vi "Lab1.vi"() -> ()   [LabVIEW 2010]
uses:
  <vilib>/measure/maspectr.llb/FFT Spectrum (Mag-Phase) for 1 Chan.vi
  <vilib>/measure/NI_MABase.lvlib
  <vilib>/measure/NI_MAPro.lvlib
  <vilib>/ptbypt/NI_PtbyPt.lvlib
panel:
  out "Power Ratio":dbl
  out "Baseband Signal (Time)":waveform(dbl)(graph)
  out "Baseband Signal (frequency)":cluster{"f0":dbl, "df":dbl, "magnitude":dbl[]}(graph)
  out "Modulated Signal (frequency)":cluster{"f0":dbl, "df":dbl, "magnitude":dbl[]}(graph)
  in  "stop":bool
  in  "Modulation Index":dbl(slide)=1.0 scale=0.0..1.0
  in  "Modulation Freq":dbl(slide)=10.0 scale=0.0..1000.0
  in  "Carrier Freq":dbl(slide)=10.0 scale=0.0..500000.0
  out "Modulated Signal (Time)":waveform(dbl)(graph)
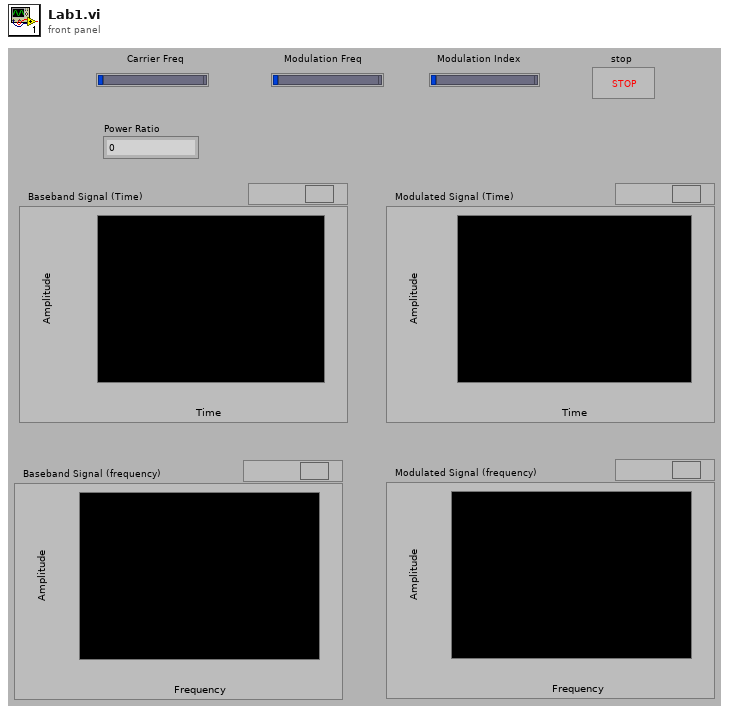
[diagram p1: front panel]
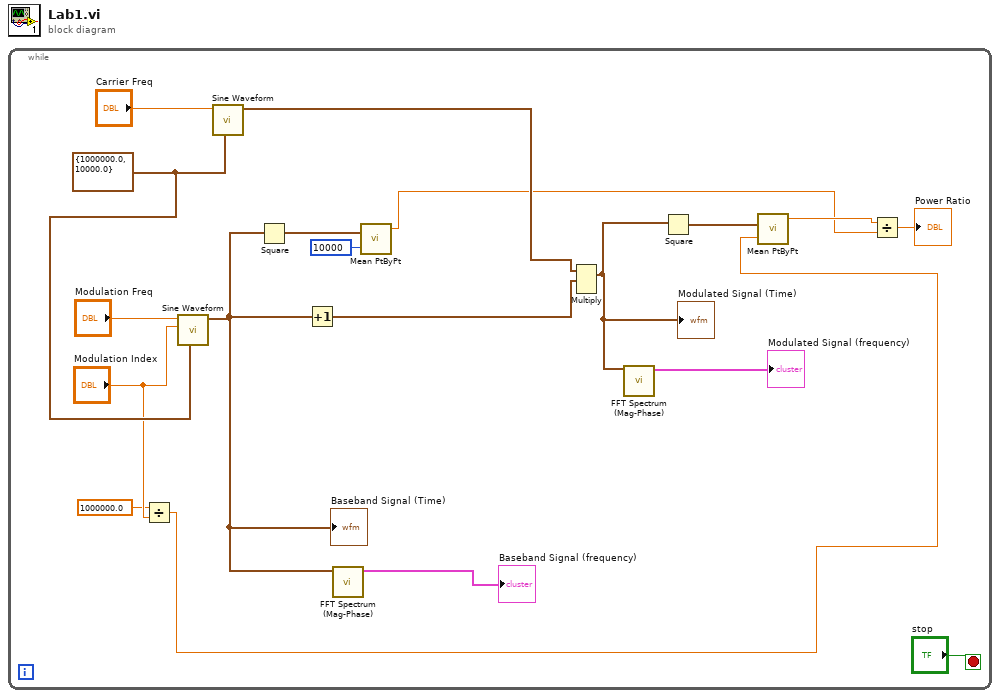
[diagram p0: block diagram]
diagram:
  n1 = while {
    stop <- "stop" stop-if-true
    w14 = cluster{"Fs":dbl, "#s":dbl} {"Fs"=1000000.0, "#s"=10000.0} ("sampling info")
    n2 = Divide(x=1000000.0, y="Modulation Index") -> (x/y=w6:dbl)
    n3 = call <vilib>:"Sine Waveform.vi"("sampling info"=w14, "amplitude"="Modulation Index", "frequency"="Modulation Freq") -> ("signal out"=w3:waveform(dbl))  [unwired: 7 in, 1 out]
    "Baseband Signal (Time)" <- w3
    n4 = call <vilib>:"Sine Waveform.vi"("sampling info"=w14, "frequency"="Carrier Freq") -> ("signal out"=w13:waveform(dbl))  [unwired: 8 in, 1 out]
    n5 = Square(x=w3) -> (x^2=w4:waveform(dbl))
    n6 = Increment(x=w3) -> (x+1=w5:waveform(dbl))
    n7 = call-poly <vilib>:"FFT Spectrum (Mag-Phase).vi"("time signal"=w3) -> ("magnitude"=→"Baseband Signal (frequency)":cluster{"f0":dbl, "df":dbl, "magnitude":dbl[]})  [unwired: 6 in, 4 out]
    n8 = call <vilib>:"Mean PtByPt.vi"("x"=w4, "sample length"=10000) -> ("mean"=w7:dbl)  [unwired: 2 in, 1 out]
    n9 = Multiply(1:w5, 2:w13) -> (0:w1:waveform(dbl))  [unwired: 1 in, 1 out]
    "Modulated Signal (Time)" <- w1
    n10 = call-poly <vilib>:"FFT Spectrum (Mag-Phase).vi"("time signal"=w1) -> ("magnitude"=→"Modulated Signal (frequency)":cluster{"f0":dbl, "df":dbl, "magnitude":dbl[]})  [unwired: 6 in, 4 out]
    n11 = Square(x=w1) -> (x^2=w2:waveform(dbl))
    n12 = call <vilib>:"Mean PtByPt.vi"("x"=w2, "sample length"=w6) -> ("mean"=w8:dbl)  [unwired: 2 in, 1 out]
    n13 = Divide(x=w8, y=w7) -> (x/y=→"Power Ratio":dbl)
  }
